vi "Fill block memory with Input Array.vi"(10 "Message In":u8[](array[numeric])=[0, 0, 0, 0, 0, 0, 0, 0, 0, 0, 0, 0, 0, 0, 0, 0, 0, 0, 0, 0, 0, 0, 0, 0, 0, 0, 0, 0, 0, 0, 0, 0, 0, 0, 0, 0, 0, 0, 0, 0, 0, 0, 0, 0, 0, 0, 0, 0, 0, 0, 0, 0, 0, 0, 0, 0, 0, 0, 0, 0, 0, 0, 0, 0, 0, 0, 0, 0, 0, 0, 0, 0, 0, 0, 0, 0, 0, 0, 0, 0, 0, 0, 0, 0, 0, 0, 0, 0, 0, 0, 0, 0, 0, 0, 0, 0, 0, 0, 0, 0, 0, 0, 0, 0, 0, 0, 0, 0, 0, 0, 0, 0, 0], 11 "Block Memory Reference In":refnum<k21>) -> (1 "Boolean Array out":bool[](array[boolean]), 2 "Array Length":u8, 3 "Block Memory Reference Out":refnum<k21>)   [LabVIEW 2014]
uses:
  <vilib>/rvi/DataTransferAndStorage/Container/Common/niFpgaContainerExecOnDevCompGetState.vi
  <vilib>/rvi/Emulation/niFpgaEmulationIsFPGAContextNoSignature.vi
  <vilib>/rvi/DataTransferAndStorage/Container/Common/niFpgaContainerGetUniqueNameForEmu.vi
  <vilib>/rvi/Emulation/niFpgaProcessEmulError.vi
  <vilib>/rvi/Emulation/niFpgaSctlEmulationGetInTimedLoop.vi
  <vilib>/rvi/errors/nirviReportUnexpectedCaseInternalError (U32).vi
  <vilib>/rvi/Memory/Memory_Emulation/niFpgaMemoryEmulationCacheClearOnFirstRun.vi
  <vilib>/rvi/Memory/Memory_Emulation/nirvimemoryEmulationManagerCache_MakeExclusive.vi
  <vilib>/rvi/Memory/Memory_Emulation/niFpgaMemoryEmulationValidateCache.vi
  <vilib>/rvi/Memory/Memory_Emulation/nirvimemoryEmulationManagerCache_InsertValue.vi
  <vilib>/Utility/error.llb/Clear Errors.vi
  <vilib>/rvi/Memory/Memory_Emulation/nirvimemoryEmulationManagerCache_ReleaseExclusive.vi
  <vilib>/rvi/Memory/Memory_Emulation/nirvimemoryEmulationManagerCache_GetValue.vi
  <vilib>/rvi/Memory/Memory_Emulation/nirvimemoryEmulationManagerCache_SetValue.vi
  <vilib>/rvi/Emulation/niFpgaSctlEmulationResourceMgr.vi
  <vilib>/rvi/DataTransferAndStorage/Container/XNode/niFpgaContainer.xnode
  <vilib>/rvi/Memory/Memory_Emulation/niFpgaMemoryEmulationRefIn.vi
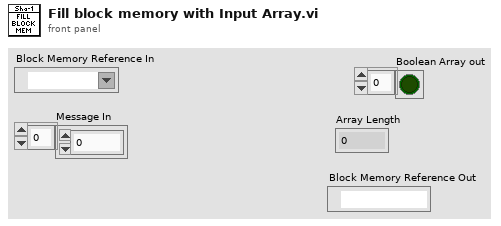
[diagram p1: front panel]
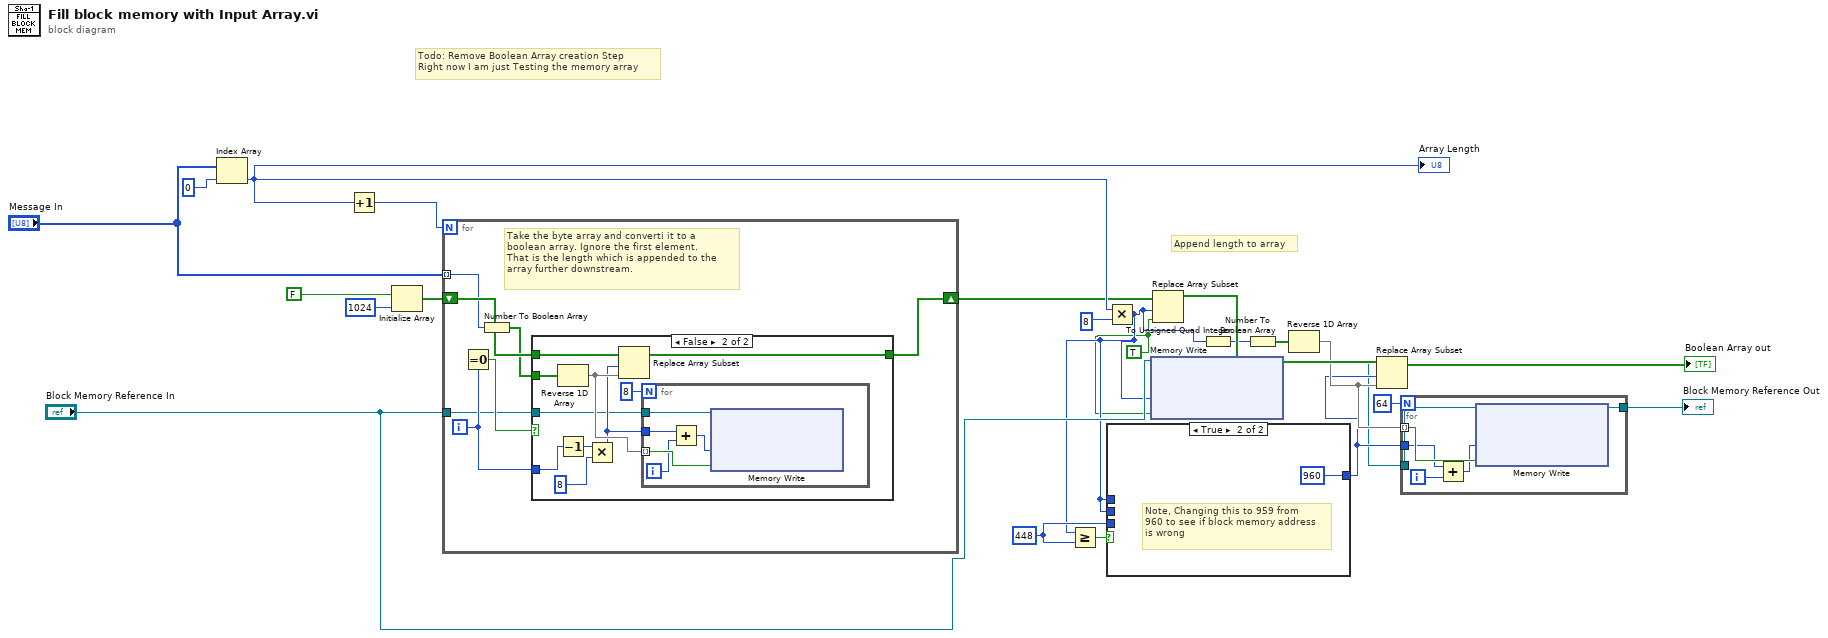
[diagram p0: block diagram]
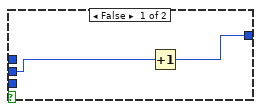
[diagram p2: hidden frame]
diagram:
  w20 = 448 ("y")
  w2 = TRUE
  # "Todo: Remove Boolean Array creation Step\nRight now I am just Testing the memory array"
  # "Append length to array"
  n1 = Index Array(array="Message In", index=0) -> (element=w21:u8)
  "Array Length" <- w21
  n2 = Increment(x=w21) -> (x+1=w16:u8)
  n3 = Initialize Array(FALSE, 1024 ("dimension size")) -> (w17:bool[])
  n4 = for {
    N: w16 -> [_]
    shift-right: [w30] -> w18
    shift-left: w17 -> [w29]
    tunnel: "Message In" -> [w25] mode=indexing
    tunnel: "Block Memory Reference In" -> [w24]
    i -> [w26]
    # "Take the byte array and converti it to a \nboolean array. Ignore the first element.\nThat is the length which is appended to the \narray further downstream."
    n5 = Equal To 0?(x=w26) -> (x = 0?=w27:bool)
    n6 = Number To Boolean Array(number=w25) -> (Boolean array=w28:bool[])
    n7 = case shown="False" w27 {
      tunnel: [w31 w41] -> w30
      tunnel: w29 -> [w31 w37]
      tunnel: w28 -> [_ w36]
      tunnel: w26 -> [_ w38]
      tunnel: w24 -> [_ w32]
      frame True {
      }
      frame False {
        n8 = Reverse 1D Array(array=w36) -> (reversed array=w34:bool[])
        n9 = Decrement(x=w38) -> (x-1=w39:i32)
        n10 = Multiply(x=w39, y=8) -> (x*y=w33:i32)
        n11 = Replace Array Subset(array=w37, new element=w34, index=w33) -> (w41:bool[])
        n12 = for {
          N: 8 -> [_]
          tunnel: w34 -> [w46] mode=indexing
          tunnel: w33 -> [w45]
          tunnel: w32 -> [w42]
          i -> [w44]
          n13 = Add(x=w45, y=w44) -> (x+y=w43:i32)
          n14 = xnode "Memory Write"("Address"=w43, "Data"=w46, "Memory In"=w42) -> ()  [unwired: 1 out]
        }
      }
    }
  }
  n15 = Multiply(x=w21, y=8) -> (x*y=w3:i32)
  n16 = Greater Or Equal?(x=w3, y=w20) -> (x >= y?=w19:bool)
  n17 = case shown="True" w19 {
    tunnel: [w47 960 ("y")] -> w6
    tunnel: w20 -> [_ _]
    tunnel: w3 -> [w48 _]
    tunnel: w3 -> [_ _]
    frame False {
      n18 = Increment(x=w48) -> (x+1=w47:i32)
    }
    frame True {
      # "Note, Changing this to 959 from\n960 to see if block memory address\nis wrong"
    }
  }
  n19 = xnode "Memory Write"("Address"=w3, "Data"=w2, "Memory In"="Block Memory Reference In") -> ("Memory Out"=w1:refnum<k21>)
  n20 = Replace Array Subset(array=w18, new element=w2, index=w3) -> (w15:bool[])
  n21 = To Unsigned Quad Integer(1:w3) -> (0:w7:u64)
  n22 = Number To Boolean Array(number=w7) -> (Boolean array=w22:bool[])
  n23 = Reverse 1D Array(array=w22) -> (reversed array=w10:bool[])
  n24 = Replace Array Subset(array=w15, new element=w10, index=w6) -> (→"Boolean Array out":bool[])
  n25 = for {
    N: 64 -> [_]
    tunnel: w1 -> [w55]
    tunnel: w6 -> [w51]
    tunnel: w10 -> [w54] mode=indexing
    tunnel: [w53] -> w8
    i -> [w52]
    n26 = Add(x=w51, y=w52) -> (x+y=w50:i32)
    n27 = xnode "Memory Write"("Address"=w50, "Data"=w54, "Memory In"=w55) -> ("Memory Out"=w53:refnum<k21>)
  }
  "Block Memory Reference Out" <- w8
